vi "Write execution period (ms).vi"(8 "error in":errorcluster, 10 "execution period (ms)":i32, 11 "Asynchronous Component Configuration in":refnum<class "asynchronous execution module configuration.lvclass">) -> (0 "error out":errorcluster, 3 "Asynchronous Component Configuration out":refnum<class "asynchronous execution module configuration.lvclass">)   [LabVIEW 2013, in "asynchronous execution module configuration.lvclass"]
doc: "Writes the <b>execution period</b> property which determines the maximum rate at which the stored component can be executed."
uses:
  asynchronous execution module configuration.lvclass
  asynchronous execution module configuration.lvclass/asynchronous execution module configuration.ctl
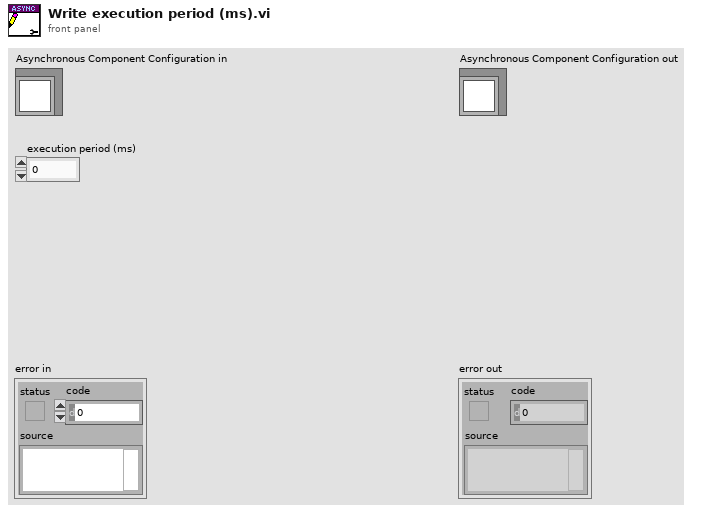
[diagram p1: front panel]
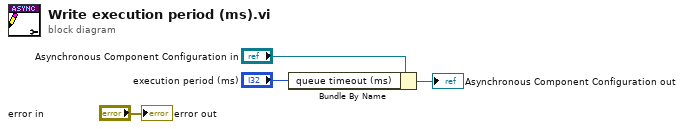
[diagram p0: block diagram]
diagram:
  n1 = Bundle By Name(cluster="Asynchronous Component Configuration in", "queue timeout (ms)"="execution period (ms)") -> (→"Asynchronous Component Configuration out":refnum<class "asynchronous execution module configuration.lvclass">)
  "error out" <- "error in"
